vi "Seven_Segment_Counter.vi"() -> ()   [LabVIEW 2022 SP3]
panel:
  out "E":bool
  out "C":bool
  out "F":bool
  out "G":bool
  out "B":bool
  out "D":bool
  out "A":bool
  # "Seven_Segment_Counter:\nProgram will continuously count from 0-9"
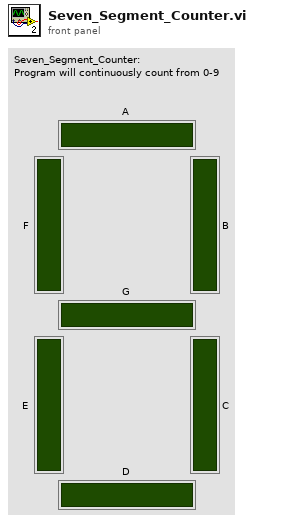
[diagram p1: front panel]
types:
  T1 = cluster{bool, bool, bool, bool, bool, bool, bool}
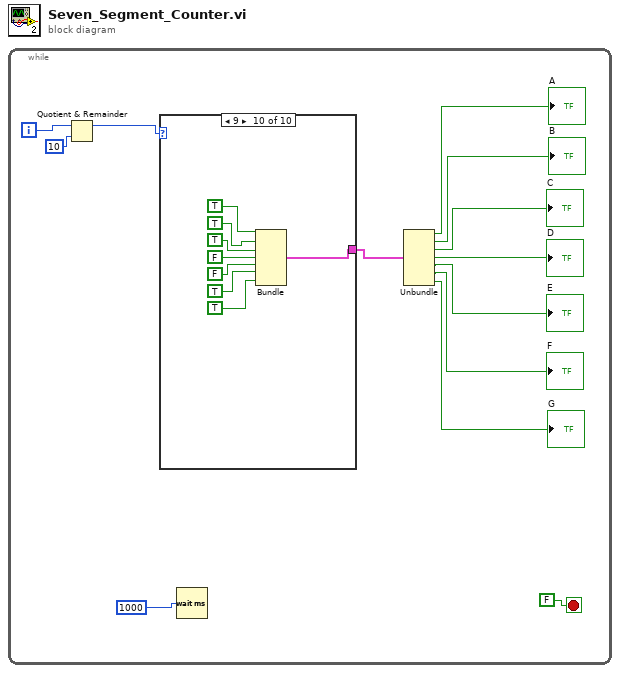
[diagram p0: block diagram]
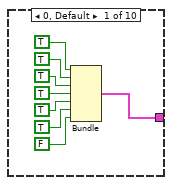
[diagram p2: hidden frame]
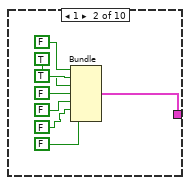
[diagram p3: hidden frame]
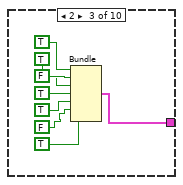
[diagram p4: hidden frame]
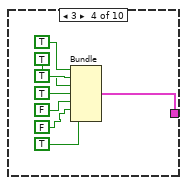
[diagram p5: hidden frame]
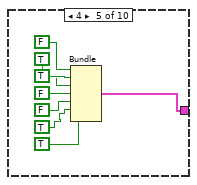
[diagram p6: hidden frame]
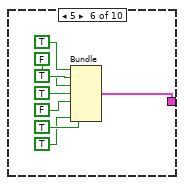
[diagram p7: hidden frame]
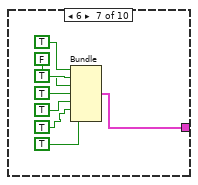
[diagram p8: hidden frame]
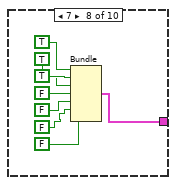
[diagram p9: hidden frame]
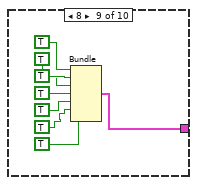
[diagram p10: hidden frame]
diagram:
  n1 = while {
    i -> [w13]
    stop <- FALSE stop-if-true
    n2 = Quotient & Remainder(x=w13, y=10) -> (x-y*floor(x/y)=w11:i32)  [unwired: 1 out]
    n3 = case shown="9" w11 {
      tunnel: [w14 w22 w30 w38 w46 w54 w62 w70 w78 w93] -> w10
      frame 0, Default {
        n4 = Bundle(TRUE, TRUE, TRUE, TRUE, TRUE, TRUE, FALSE) -> (w14:T1)  [unwired: 1 in]
      }
      frame 1 {
        n5 = Bundle(FALSE, TRUE, TRUE, FALSE, FALSE, FALSE, FALSE) -> (w22:T1)  [unwired: 1 in]
      }
      frame 2 {
        n6 = Bundle(TRUE, TRUE, FALSE, TRUE, TRUE, FALSE, TRUE) -> (w30:T1)  [unwired: 1 in]
      }
      frame 3 {
        n7 = Bundle(TRUE, TRUE, TRUE, TRUE, FALSE, FALSE, TRUE) -> (w38:T1)  [unwired: 1 in]
      }
      frame 4 {
        n8 = Bundle(FALSE, TRUE, TRUE, FALSE, FALSE, TRUE, TRUE) -> (w46:T1)  [unwired: 1 in]
      }
      frame 5 {
        n9 = Bundle(TRUE, FALSE, TRUE, TRUE, FALSE, TRUE, TRUE) -> (w54:T1)  [unwired: 1 in]
      }
      frame 6 {
        n10 = Bundle(TRUE, FALSE, TRUE, TRUE, TRUE, TRUE, TRUE) -> (w62:T1)  [unwired: 1 in]
      }
      frame 7 {
        n11 = Bundle(TRUE, TRUE, TRUE, FALSE, FALSE, FALSE, FALSE) -> (w70:T1)  [unwired: 1 in]
      }
      frame 8 {
        n12 = Bundle(TRUE, TRUE, TRUE, TRUE, TRUE, TRUE, TRUE) -> (w78:T1)  [unwired: 1 in]
      }
      frame 9 {
        n13 = Bundle(TRUE, TRUE, TRUE, FALSE, FALSE, TRUE, TRUE) -> (w93:T1)  [unwired: 1 in]
      }
    }
    n14 = Wait (ms)(milliseconds to wait=1000) -> ()  [unwired: 1 out]
    n15 = Unbundle(w10) -> (→"A":bool, →"B":bool, →"C":bool, →"D":bool, →"E":bool, →"F":bool, →"G":bool)
  }
